vi "Write Configuration Dictionary.vi"(8 "error in (no error)":errorcluster, 10 "Configuration Dictionary":variant, 11 "ITestSettings in":refnum<class "ITestSettings.lvclass">) -> (0 "error out":errorcluster, 3 "ITestSettings out":refnum<class "ITestSettings.lvclass">)   [LabVIEW 2016, in "ITestSettings.lvlib" / "ITestSettings.lvclass"]
uses:
  ITestSettings.lvclass
  ITestSettings.lvclass/ITestSettings.ctl
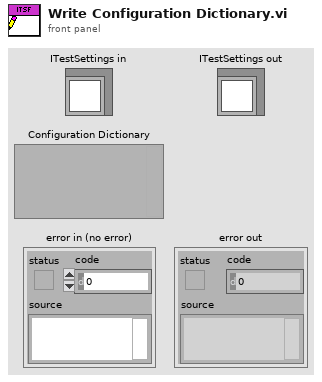
[diagram p1: front panel]
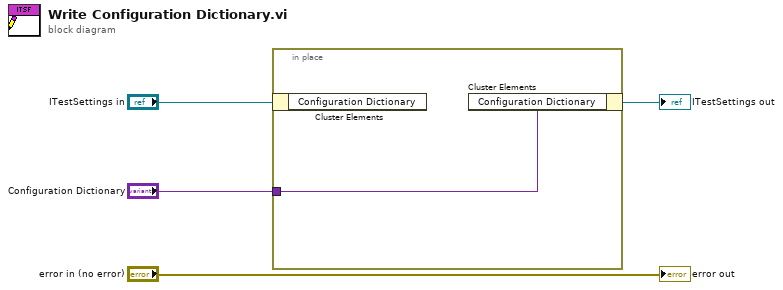
[diagram p0: block diagram]
diagram:
  n1 = in-place {
    in-place-border: "Configuration Dictionary" -> [w5]
    n2 = in-place-cluster #1("ITestSettings in") -> ()  [unwired: 1 out]
    n3 = in-place-cluster #1("Configuration Dictionary"=w5) -> (→"ITestSettings out":refnum<class "ITestSettings.lvclass">)
  }
  "error out" <- "error in (no error)"
